vi "循环采样.vi"(10 "reference输入":refnum<vi>, 11 "Array输入":refnum<vi>) -> (3 "测量序列":dbl[](array[numeric]))   [LabVIEW 2016]
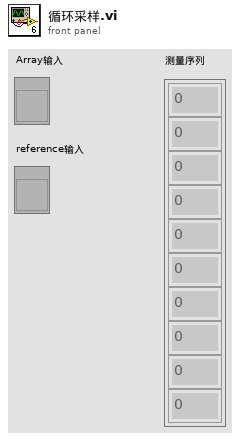
[diagram p1: front panel]
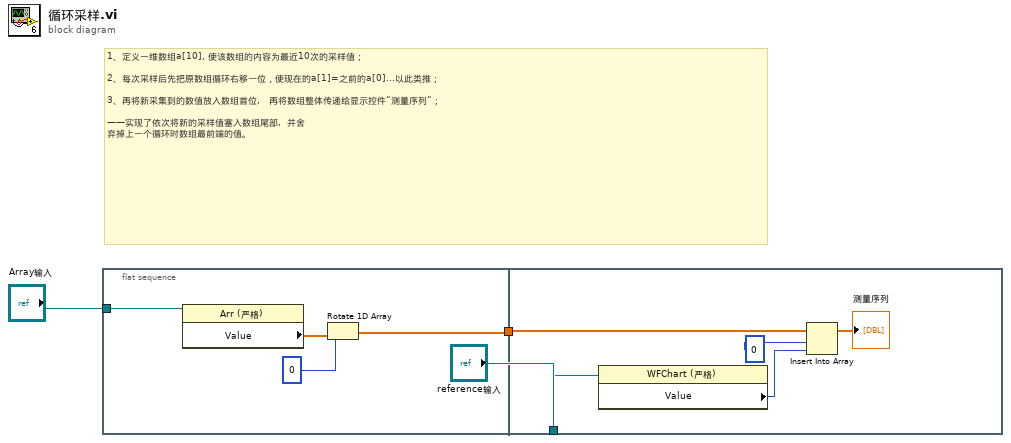
[diagram p0: block diagram]
diagram:
  # "1、定义一维数组a[10], 使该数组的内容为最近10次的采样值；\n\n2、每次采样后先把原数组循环右移一位，使现在的a[1]=之前的a[0]...以此类推；\n\n3、再将新采集到的数值放入数组首位,   再将数组整体传递给显示控件“测量序列“；\n\n——实现了依次将新的采样值塞入数组尾部,  并舍\n弃掉上一个循环时数组最前端的值。"
  n1 = flat-sequence {
    tunnel: [w6] -> w3
    tunnel: "Array输入" -> [w4]
    tunnel: w3 -> [w11]
    tunnel: "reference输入" -> [w10]
    frame #0 {
      n2 = property class="Arr (严格)"(reference=w4) -> ("Value"=w7:dbl[])  [unwired: 1 in, 2 out]
      n3 = Rotate 1D Array(1:w7, 2:0 ("n")) -> (0:w6:dbl[])
    }
    frame #1 {
      n4 = property class="WFChart (严格)"(reference=w10) -> ("Value"=w9:i32)  [unwired: 1 in, 2 out]
      n5 = Insert Into Array(array=w11, index=0 ("索引"), new element=w9) -> (→"测量序列":dbl[])
    }
  }
